vi "scanTrigger.vi"() -> (14 "triggeredScan":bool)   [LabVIEW 2014]
uses:
  Sequencer/sequencerGlobVars.vi
  scanTriggerGlobalVars.vi
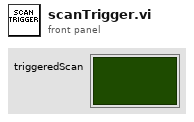
[diagram p1: front panel]
types:
  T1 = typedef "triggerTypes.ctl" = enum16{"noTrigger", "singleHitDelay", "singleHit", "software", "sweep"}
  T2 = typedef "selectTrigger.ctl" = enum8{"Ext0", "Ext1", "Ext2", "Ext3", "Ext4", "Ext5", "Ext6", "Ext7", "Int0", "Int1", "Int2", "Int3", "Int4", "Int5", "Int6", "Int7"}
  T3 = typedef "triggerEdge.ctl" = enum8{"either", "false-true", "true-false"}
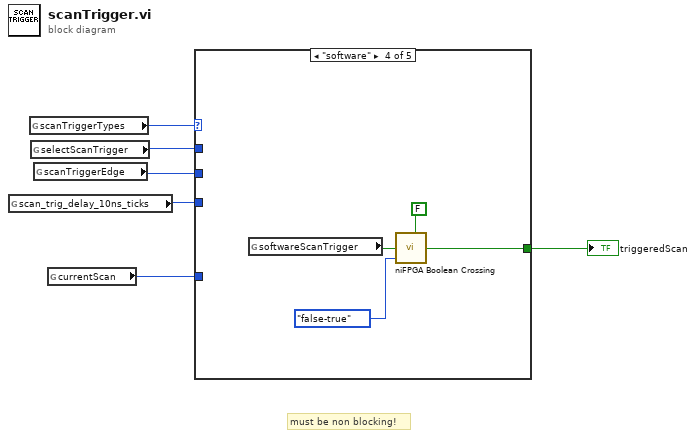
[diagram p0: block diagram]
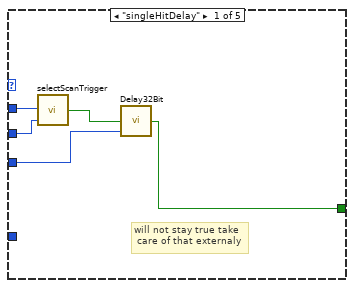
[diagram p2: hidden frame]
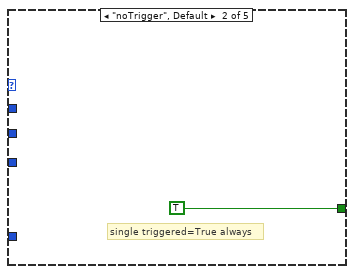
[diagram p3: hidden frame]
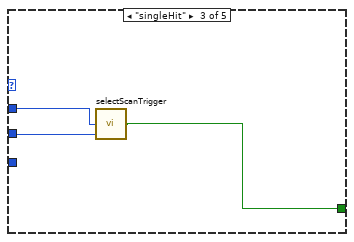
[diagram p4: hidden frame]
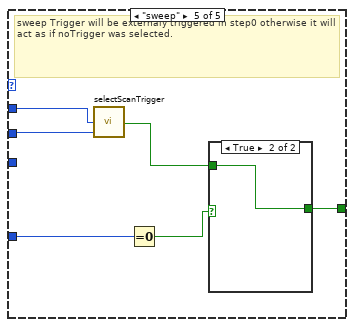
[diagram p5: hidden frame]
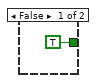
[diagram p6: hidden frame]
diagram:
  # "must be non blocking!"
  n1 = global read "scanTriggerGlobalVars.vi" "scan_trig_delay_10ns_ticks"() -> (w4:u32)
  n2 = global read "scanTriggerGlobalVars.vi" "scanTriggerTypes"() -> (w1:T1)
  n3 = global read "scanTriggerGlobalVars.vi" "selectScanTrigger"() -> (w2:T2)
  n4 = global read "scanTriggerGlobalVars.vi" "scanTriggerEdge"() -> (w3:T3)
  n5 = global read "sequencerGlobVars.vi" "currentScan"() -> (w5:i32)
  n6 = case shown="\"software\"" w1 {
    tunnel: w2 -> [w8 _ w14 _ w21]
    tunnel: w4 -> [w11 _ _ _ _]
    tunnel: [w10 TRUE w15 w19 w23] -> w6
    tunnel: w3 -> [w7 _ w13 _ w20]
    tunnel: w5 -> [_ _ _ _ w25]
    frame "singleHitDelay" {
      # "will not stay true take\n care of that externaly"
      n7 = call "selectScanTrigger.vi"("scanTriggerEdge"=w7, "MCSSelectScanTrigger"=w8) -> ("fired"=w9:bool)  [unwired: 3 in]
      n8 = call "Delay32Bit.vi"("delay(ticks)"=w11, "In"=w9) -> ("Out"=w10:bool)  [unwired: 3 in]
    }
    frame "noTrigger", Default {
      # "single triggered=True always"
    }
    frame "singleHit" {
      n9 = call "selectScanTrigger.vi"("scanTriggerEdge"=w13, "MCSSelectScanTrigger"=w14) -> ("fired"=w15:bool)  [unwired: 3 in]
    }
    frame "software" {
      n10 = global read "scanTriggerGlobalVars.vi" "softwareScanTrigger"() -> (w16:bool)
      n11 = call <vilib>:"niFPGA Boolean Crossing.vi"("input"=w16, "direction"=enum8{"either", "false-true", "true-false"}."false-true", "initialize"=FALSE) -> ("crossing"=w19:bool)  [unwired: 6 in]
    }
    frame "sweep" {
      # "sweep Trigger will be externaly triggered in step0 otherwise it will act as if noTrigger was selected."
      n12 = call "selectScanTrigger.vi"("scanTriggerEdge"=w20, "MCSSelectScanTrigger"=w21) -> ("fired"=w22:bool)  [unwired: 3 in]
      n13 = Equal To 0?(x=w25) -> (x = 0?=w24:bool)
      n14 = case shown="True" w24 {
        tunnel: w22 -> [_ w27]
        tunnel: [TRUE ("fired") w27] -> w23
        frame False {
        }
        frame True {
        }
      }
    }
  }
  "triggeredScan" <- w6
